vi "CONTROL_PWM.vi"() -> ()   [LabVIEW 2010]
uses:
  <vilib>/Instr/_visa.llb/VISA Configure Serial Port (Instr).vi
panel:
  in  "ACTIVACION PWM":bool
  out "PWM % 2":i8(slide) caption="PWM %" scale=0.0..100.0 scale format="%#.0f"
  in  "Decena":u8 max=9 step=1 format="%#.1f"
  in  "Centena":u8 max=1 step=1 format="%#.1f"
  in  "Unidad":u8 max=9 step=1 format="%#.1f"
  in  "flow control":u16(ring) items=["None"=0, "XON/XOFF"=1, "RTS/CTS"=2, "DTR/DSR"=4]
  in  "stop bits":u16(ring)=10 items=["1.0"=10, "1.5"=15, "2.0"=20]
  in  "parity":u16(ring) items=["None", "Odd", "Even", "Mark", "Space"]
  in  "data bits":u16=8 min=5 max=8 step=1
  in  "VISA resource name":refnum<visa-resource-name>="COM1"
  in  "baud rate":u32=9600
  # "PARAMETROS PUERTO SERIAL"
  # "AJUSTE DE VALOR PWM (0 a 100)"
  # "%"
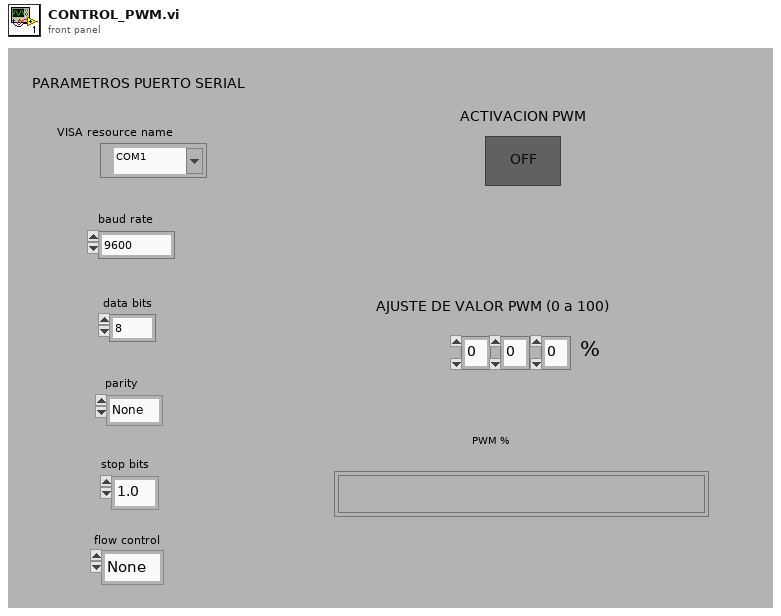
[diagram p1: front panel]
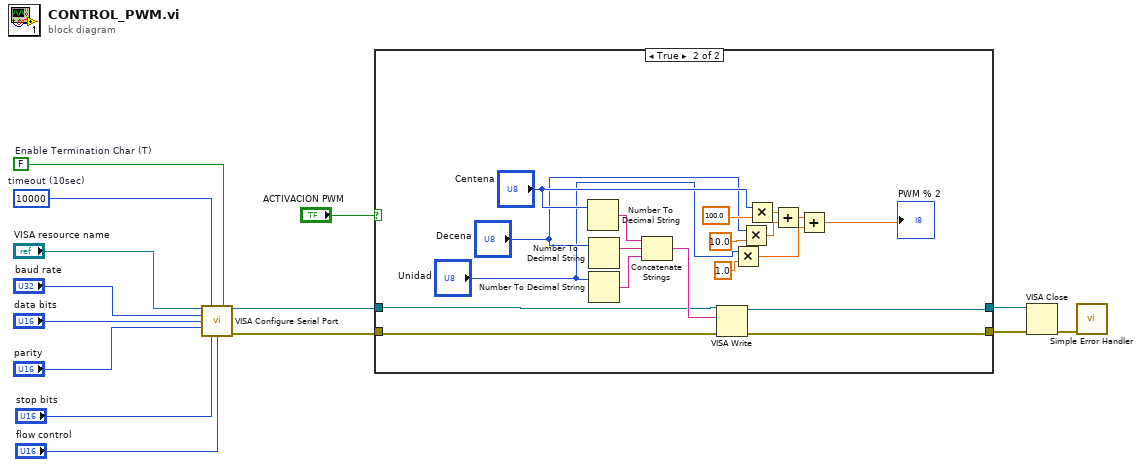
[diagram p0: block diagram]
diagram:
  w10 = FALSE  # Enable Termination Char (T)
  w11 = u32 10000  # timeout (10sec)
  n1 = call-poly "VISA Configure Serial Port"("VISA resource name"="VISA resource name", "timeout (10sec)"=w11, "Enable Termination\nChar (T)"=w10, "baud rate (9600)"="baud rate", "data bits (8)"="data bits", "parity (0:none)"="parity", "stop bits (10: 1 bit)"="stop bits", "flow control (0:none)"="flow control") -> ("VISA resource name out"=w2:refnum<visa-resource-name>, "error out"=w1:errorcluster)  [unwired: 6 in]
  n2 = case shown="True" "ACTIVACION PWM" {
    tunnel: w2 -> [w16 w20]
    tunnel: w1 -> [w15 w19]
    tunnel: [w16 w18] -> w4
    tunnel: [w15 w17] -> w3
    frame False {
    }
    frame True {
      n3 = Number To Decimal String(number="Centena") -> (decimal integer string=w33:string)  [unwired: 1 in]
      n4 = Number To Decimal String(number="Decena") -> (decimal integer string=w34:string)  [unwired: 1 in]
      n5 = Number To Decimal String(number="Unidad") -> (decimal integer string=w35:string)  [unwired: 1 in]
      n6 = Concatenate Strings(w33, w34, w35) -> (w32:string)
      n7 = VISA Write(VISA resource name=w20, write buffer=w32, error in (no error)=w19) -> (VISA resource name out=w18:refnum<visa-resource-name>, error out=w17:errorcluster)  [unwired: 1 out]
      n8 = Multiply(x="Unidad", y=1.0) -> (x*y=w27:dbl)
      n9 = Multiply(x="Decena", y=10.0) -> (x*y=w25:dbl)
      n10 = Multiply(x="Centena", y=100.0) -> (x*y=w24:dbl)
      n11 = Add(x=w24, y=w25) -> (x+y=w26:dbl)
      n12 = Add(x=w26, y=w27) -> (x+y=→"PWM % 2":dbl)
    }
  }
  n13 = VISA Close(VISA resource name=w4, error in (no error)=w3) -> (error out=w5:errorcluster)
  n14 = call <vilib>:"Simple Error Handler.vi"("error in (no error)"=w5) -> ()  [unwired: 4 in, 5 out]
